vi "Beta Ver 1.1.vi"() -> ()   [LabVIEW 2015]
uses:
  <instrlib>/Keithley 622x LV 2009/Configure/Source/Typedefs/KE622x -- Current Range.ctl
  <instrlib>/Keithley 622x LV 2009/Configure/Source/Typedefs/KE622x -- Current Ranges.ctl
  <instrlib>/Keithley 622x LV 2009/Typedefs/KE622x -- On Off Control.ctl
  <instrlib>/Keithley 622x LV 2009/Utility/Typedefs/KE622x -- Instrument Type.ctl
  <instrlib>/Keithley 622x LV 2009/Configure/Source/Typedefs/KE622x -- Voltage Limit.ctl
  <instrlib>/Keithley 2000/Public/Configure/Configure DC Volts.vi
  <userlib>/LV-Link3/PolySubVIs/DtCreateAinChan.vi
  <userlib>/LV-Link3/PolySubVIs/DtOLReadMultipleSingle.vi
  <instrlib>/Keithley 2000/Keithley 2000.lvlib
  <instrlib>/Keithley 622x LV 2009/Keithley 622x.lvlib
panel:
  in  "Setup":u16(ring) items=["START, STOP, STEP, CONFIGURATION", "PRINCETON LOCK-IN AMP"]
  out "prev_time_const":i32
  out "prev_range":i32
  out "XTC":i32
  out "SEN":i32
  in  "Time Delay":u16(ring) items=["0.1", "1", "3", "10", "30", "60"]
  out "FILE":refnum<file>
  out "Tick":u32
  in  "MULTIPLE GRAPHS Y":u16(ring) items=["Linear", "Log"]
  in  "MULTIPLE GRAPHS X":u16(ring) items=["Linear", "Log"]
  in  "TIME GRAPH Y":u16(ring) items=["Linear", "Log"]
  in  "TIME GRAPH X":u16(ring) items=["Linear", "Log"]
  in  "Lock-In, Y":dbl=1.0
  in  "Lock-In, X":dbl=1.0
  in  "DAQ A4":dbl=1.0
  in  "DAQ A3":dbl=1.0
  in  "DAQ A2":dbl=1.0
  in  "DAQ A1":dbl=1.0
  in  "DAQ A0":dbl=1.0
  in  "2000":dbl=1.0
  in  "Current":dbl=1000.0
  in  "Display Type 3":u16(ring)=3 items=["X %", "Y %", "X Calibrated", "Y Calibrated", "Mag %", "Mag Calibrated", "Phase Degrees", "Ratio", "ADC 1", "ADC 2", "ADC 3", "ADC 4 ", "Noise %", "Noise Calibrated", "Ref Frequency", "", ""]
  in  "Display Type 2":u16(ring)=2 items=["X %", "Y %", "X Calibrated", "Y Calibrated", "Mag %", "Mag Calibrated", "Phase Degrees", "Ratio", "ADC 1", "ADC 2", "ADC 3", "ADC 4 ", "Noise %", "Noise Calibrated", "Ref Frequency", "", ""]
  out "Units 3":string
  out "Display 3":dbl format="%.3f"
  out "Units 2":string
  out "Display 2":dbl format="%.3f"
  out "DAQ A4":dbl format="%#_13g"
  out "DAQ_clust":T1
  out "DAQ A3":dbl format="%#_13g"
  out "DAQ A2":dbl format="%#_13g"
  out "DAQ A1":dbl format="%#_13g"
  out "Real stop cur":dbl format="%#_13g"
  out "Real start cur":dbl format="%#_13g"
  in  "Stop cur prefix":u16(ring)=2
  in  "Start cur prefix":u16(ring)=2
  out "MULTIPLE GRAPHS":cluster{dbl[], dbl[]}[](graph)
  in  "X-Axis":T2(ring)
  in  "Range":u8(ring)=20 items=["100nV", "200nV", "500nV", "1µV", "2µV", "5µV", "10µV", "20µV", "50µV", "100µV", "200µV", "500µV", "1mV", "2mV", "5mV", "10mV", "20mV", "50mV", "100mV", "200mV", "500mV", "1V"]
  in  "Display Type copy":u16(ring)=3 items=["X %", "Y %", "X Calibrated", "Y Calibrated", "Mag %", "Mag Calibrated", "Phase Degrees", "Ratio", "ADC 1", "ADC 2", "ADC 3", "ADC 4 ", "Noise %", "Noise Calibrated", "Ref Frequency", "", ""]
  out "Units copy":string
  out "Display copy":dbl format="%.3f"
  out "Overload":bool
  out "Display":dbl format="%.3f"
  out "Units":string
  in  "Display Type":u16(ring)=2 items=["X %", "Y %", "X Calibrated", "Y Calibrated", "Mag %", "Mag Calibrated", "Phase Degrees", "Ratio", "ADC 1", "ADC 2", "ADC 3", "ADC 4 ", "Noise %", "Noise Calibrated", "Ref Frequency", "", ""]
  in  "Time Constant":u16(ring)=7 items=["MIN", "1ms", "3ms", "10ms", "30ms", "100ms", "300ms", "1s", "3s", "10s", "30s", "100s", "300s"]
  in  "Slope":u8(ring) items=["6db/octave", "12dB/octave"]
  in  "Dynamic Reserve":u16(ring)=1 items=["High Stability", "Normal", "High Reserve"]
  in  "Auto Sensitivity":bool
  in  "Auto Measure":bool
  out "6221_error_out":errorcluster
  out "2000_error_out":errorcluster
  out "5110_error_out":errorcluster
  out "Input Mode":i32(ring) items=[" Voltage Input (A or A-B) ", "Current Input 10E6 V/A", "Current Input 10E8 V/A"]
  out "5110":refnum<visa-resource-name>
  in  "GPIB Address":i8=11 min=1 max=32 step=1
  out "DAQ A0":dbl format="%#_13g"
  out "2000":dbl format="%#_13g"
  in  "Device":string(combo)
  in  "Number \nof points":i32=10
  in  "Folder\nprename":string
  out "TIME GRAPH":cluster{dbl[], dbl[]}[](graph)
  out "T0":u32
  out "LIMIT":bool
  out "LIMIT":bool
  out "Error Code":string
  in  "Comments":string
  out "2000":refnum<visa-resource-name>
  out "6221":refnum<visa-resource-name>
  out "Step  (A)":dbl=5e-05 format="%#_3p"
  in  "Stop\ncurrent (A)":dbl=2.0 format="%#_6p"
  in  "Start \ncurrent (A)":dbl=1.0 format="%#_6p"
  in  "Check For SCPI Errors? (T)":bool=TRUE
  out "Interlock Tripped?":bool
  out "Compliance?":bool
  in  "Turn Off Output \nIf Compliance?":bool=TRUE
  in  "Turning ON/OFF\ncurrent output":T3=enum."On"
  in  "Range Selection":T4={"Auto Range?"=TRUE, "Man / Selected\nRange"=enum."2nA"}
  # "FILE CONFIGURATION"
  # "ADMIN PANEL"
  # "MULTIPLIERS"
  # "SCALES"
  # "KEITHLEY 6221 CONFIGURATION (ADMIN ONLY)"
  # "KEITHLEY DAQ CONFIGURATION (ADMIN ONLY)"
  # "PRINCETON LOCK-IN AMP (ADMIN ONLY)"
  # "I don't know what the hell it is,\njust don't touch it"
  # "INPUT CONFIGURATION"
  # "READINGS"
  # "IF ON"
  # "Compliance = Limiting output voltage\nThis switch determines if we want to switch \noff the current output if wee exceed compliance"
  # "SCALES"
  # "There is a safe switch at \nthe back of the instrument \nThis indicator shows if it is on"
  # "You have hit a damn jackpot \nby exceeding the limited voltage\nCongrats"
  # "LOCK-IN READINGS"
  # "RIGHT DISPLAY"
  # "LEFT DISPLAY"
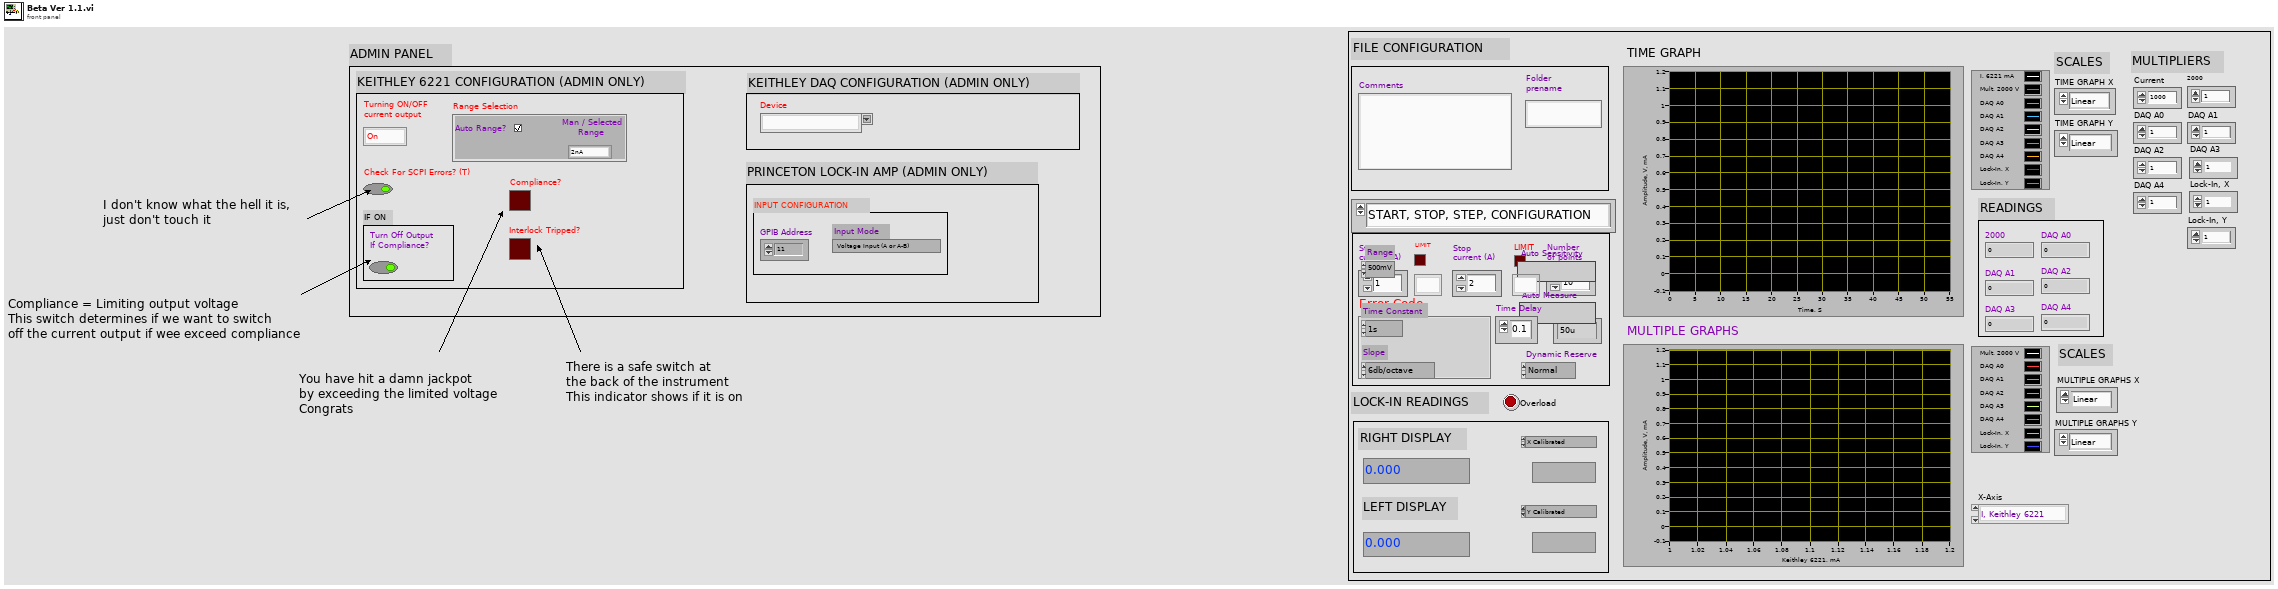
[diagram p1: front panel]
types:
  T1 = cluster{"Task out":i32, "Actual Number of Channels":u32, "error out":errorcluster}
  T2 = enum16{"I, Keithley 6221", "V, Keithley 2000", "V, Keithley DAQ A0", "V, Keithley DAQ A1", "V, Keithley DAQ A2", "V, Keithley DAQ A3", "V, Keithley DAQ A4", "V, Lock-In X", "V, Lock-In Y"}
  T3 = typedef "Keithley 622x.lvlib/KE622x -- On Off Control.ctl" = enum16{"Off", "On"}
  T4 = typedef "Keithley 622x.lvlib/KE622x -- Current Range.ctl" = cluster{"Auto Range?":bool, "Man / Selected\nRange":T5}
  T5 = typedef "Keithley 622x.lvlib/KE622x -- Current Ranges.ctl" = enum16{"2nA", "20nA", "200nA", "2uA", "20uA", "200uA", "2mA", "20mA", "100mA"}
  T6 = typedef "Keithley 622x.lvlib/KE622x -- Instrument Type.ctl" = enum16{"KE6220", "KE6221"}
  T7 = typedef "Keithley 622x.lvlib/KE622x -- Voltage Limit.ctl" = dbl
  T8 = cluster{dbl[], dbl[], dbl[], dbl[], dbl[], dbl[], dbl[], dbl[], dbl[], dbl[]}
  T9 = cluster{"5110":refnum<visa-resource-name>, "2000":refnum<visa-resource-name>, "6221":refnum<visa-resource-name>, "5110_error_out":errorcluster, "6221_error_out":errorcluster, "2000_error_out":errorcluster, "DAQ_clust":cluster{"Task out":i32, "Actual Number of Channels":u32, "error out":errorcluster}}
  T10 = cluster{dbl, dbl, dbl, dbl, dbl, "Measurement":dbl}
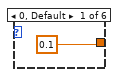
[diagram p2: hidden frame]
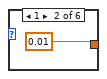
[diagram p3: hidden frame]
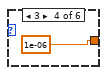
[diagram p4: hidden frame]
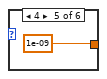
[diagram p5: hidden frame]
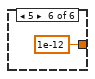
[diagram p6: hidden frame]
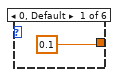
[diagram p7: hidden frame]
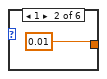
[diagram p8: hidden frame]
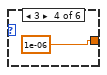
[diagram p9: hidden frame]
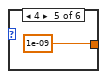
[diagram p10: hidden frame]
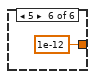
[diagram p11: hidden frame]
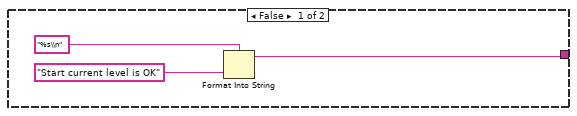
[diagram p12: hidden frame]
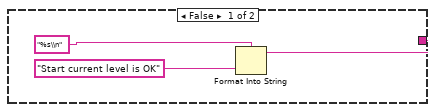
[diagram p13: hidden frame]
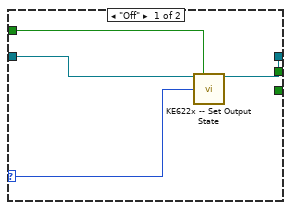
[diagram p14: hidden frame]
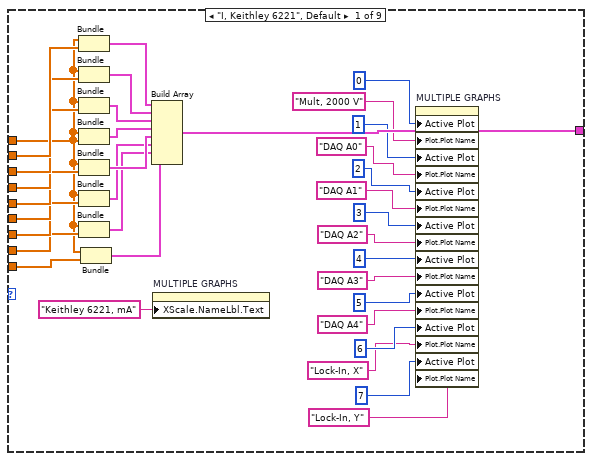
[diagram p15: hidden frame]
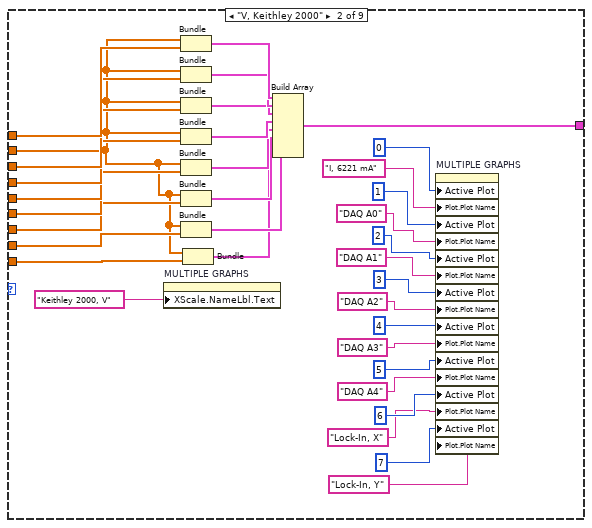
[diagram p16: hidden frame]
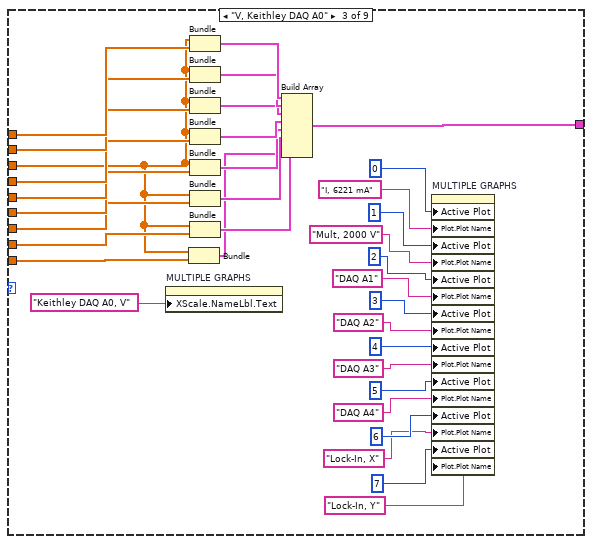
[diagram p17: hidden frame]
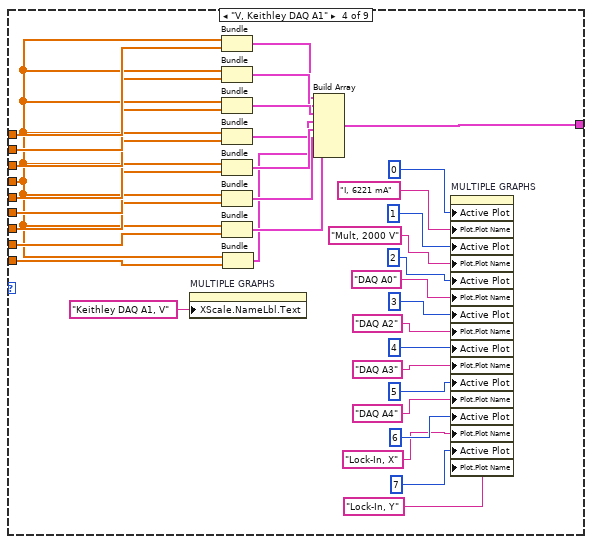
[diagram p18: hidden frame]
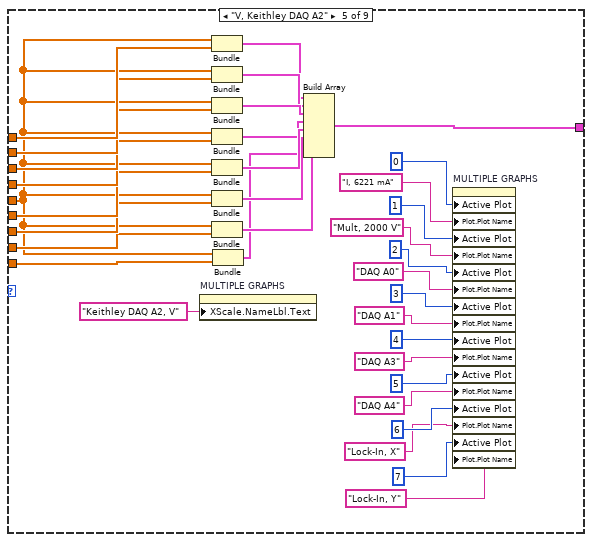
[diagram p19: hidden frame]
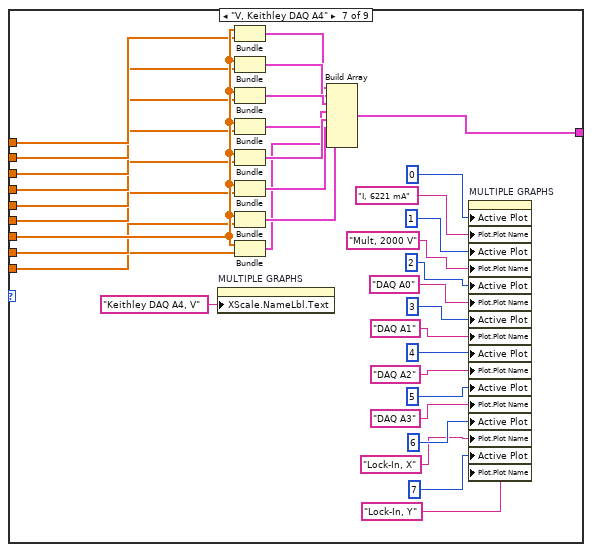
[diagram p20: hidden frame]
diagram:
  n1 = flat-sequence {
    tunnel: [w153] -> w1
    tunnel: w1 -> [w942]
    frame #0 {
      w16 = TRUE  # reset
      w17 = FALSE  # ID query
      # "Initialize Keithley DAQ \n(getting board name)"
      # "Initialize Lock-In 5110"
      # "Initialize Keithley 2000"
      # "Initialize Keithley 6221"
      n2 = call <userlib>:"DtOLGetBoardNames.vi"() -> ("Number of boards"=w2:u32)  [unwired: 9 in, 2 out]
      n3 = Initialize Array("", w2) -> (w4:string[])
      n4 = call <instrlib>:"Initialize.vi"("VISA resource name"=refnum<visa-resource-name> "KEITHLEY_MULTIMETER") -> ("VISA resource name out"=w12:refnum<visa-resource-name>)  [unwired: 17 in, 1 out]
      n5 = for {
        N: w2 -> [_]
        shift-right: [w26] -> w7
        shift-left: w4 -> [w27]
        i -> [w25]
        n6 = Add(x=1, y=w25) -> (x+y=w29:i32)
        n7 = call <userlib>:"DtOLGetBoardNames.vi"("Select Board"=w29) -> ("Board Name"=w24:string)  [unwired: 8 in, 2 out]
        n8 = Replace Array Subset(array=w27, new element=w24, index=w25) -> (w26:string[])
      }
      n9 = call <instrlib>:"Initialize.vi"("VISA resource name"=refnum<visa-resource-name> "KEITHLEY_DC_AC_CURRENT_SOURCE", "Error Queue Option"=enum16{"Clear Error Queue", "Error Query"}."Clear Error Queue", "Instrument Type"=KE622x_--_Instrument_Type."KE6221") -> ("VISA resource name out"=→"6221":refnum<visa-resource-name>, "error out"=→"6221_error_out":errorcluster)  [unwired: 11 in]
      n10 = call-poly <instrlib>:"Configure Measurement.vi"("VISA resource name"=w12) -> ("VISA resource name out"=→"2000":refnum<visa-resource-name>, "error out"=→"2000_error_out":errorcluster)  [unwired: 17 in]
      n11 = call "SR51XX Initialize"("VISA session (for class)"=refnum<visa-resource-name> "LOCK_IN_5110_PRINCETON", "Interface"=FALSE, "ID query"=w17, "GPIB Address"="GPIB Address", "reset"=w16) -> ("VISA session"=→"5110":refnum<visa-resource-name>, "error out"=→"5110_error_out":errorcluster)  [unwired: 8 in, 1 out]
      n12 = Index Array(array=w7, index=0) -> (element=w6:string)
      n13 = property on="Device" class="CmbBox"("Strings[]"=w7, "Value"=w6) -> ()  [unwired: 2 in, 2 out]
    }
    frame #1 {
      # "Putting in a loop \ninstead of \"STOP\""
      n14 = case shown="2" "Start cur prefix" {
        tunnel: [0.1 0.01 0.001 1e-06 1e-09 1e-12] -> w39
        frame 0, Default {
        }
        frame 1 {
        }
        frame 2 {
        }
        frame 3 {
        }
        frame 4 {
        }
        frame 5 {
        }
      }
      n15 = case shown="2" "Stop cur prefix" {
        tunnel: [0.1 0.01 0.001 1e-06 1e-09 1e-12] -> w41
        frame 0, Default {
        }
        frame 1 {
        }
        frame 2 {
        }
        frame 3 {
        }
        frame 4 {
        }
        frame 5 {
        }
      }
      n16 = Multiply(x=w39, y="Start \ncurrent (A)") -> (x*y=w43:dbl)
      "Real start cur" <- w43
      n17 = Multiply(x=w41, y="Stop\ncurrent (A)") -> (x*y=w44:dbl)
      "Real stop cur" <- w44
      n18 = Greater?(x=w44, y=T7 0.01) -> (0:w33:bool)
      n19 = Greater?(x=w43, y=T7 0.01) -> (0:w34:bool)
      n20 = case shown="True" w33 {
        selector: w33 -> [_ w60]
        tunnel: [w57 w63] -> w31
        frame False {
          n21 = Format Into String(format string="%s\\n", "Start current level is OK" ("false string")) -> (resulting string=w57:string)  [unwired: 2 in, 1 out]
        }
        frame True {
          n22 = flat-sequence {
            tunnel: [w65] -> w62
            tunnel: [w64] -> w61
            tunnel: w60 -> [w64]
            tunnel: [w69] -> w63
            tunnel: w62 -> [w69]
            tunnel: w61 -> [w70]
            frame #0 {
              n23 = Format Into String(format string="%s\\n%s\\n", "Stop current level" ("String"), "exceeded the  limit: 10mA" ("input 2")) -> (resulting string=w65:string)  [unwired: 2 in, 1 out]
            }
            frame #1 {
              n24 = while {
                tunnel: w70 -> [w71]
                stop <- w71 continue-if-true
                "LIMIT" <- w71
              }
              n25 = property on="Error Code" class="Str"("Text.Text"=w69) -> ()  [unwired: 2 in, 2 out]
            }
          }
        }
      }
      n26 = case shown="True" w34 {
        selector: w34 -> [_ w76]
        tunnel: [w72 w78] -> w32
        frame False {
          n27 = Format Into String(format string="%s\\n", "Start current level is OK" ("false string")) -> (resulting string=w72:string)  [unwired: 2 in, 1 out]
        }
        frame True {
          n28 = flat-sequence {
            tunnel: [w80] -> w77
            tunnel: w76 -> [w79]
            tunnel: [w79] -> w75
            tunnel: [w84] -> w78
            tunnel: w77 -> [w84]
            tunnel: w75 -> [w85]
            frame #0 {
              n29 = Format Into String(format string="%s\\n%s\\n", "Start current level" ("String"), "exceeded the limit: 10mA" ("input 2")) -> (resulting string=w80:string)  [unwired: 2 in, 1 out]
            }
            frame #1 {
              n30 = while {
                tunnel: w85 -> [w86]
                stop <- w86 continue-if-true
                "LIMIT" <- w86
              }
              n31 = property on="Error Code" class="Str"("Text.Text"=w84) -> ()  [unwired: 2 in, 2 out]
            }
          }
        }
      }
      n32 = Concatenate Strings(w32, w31) -> (→"Error Code":string)
    }
    frame #2 {
      # "Calculating steps by number\nof points"
      n33 = local read "Real stop cur"() -> (w88:dbl)
      n34 = local read "Real start cur"() -> (w89:dbl)
      n35 = Subtract(x=w88, y=w89) -> (x-y=w91:dbl)
      n36 = Divide(x=w91, y="Number \nof points") -> (x/y=→"Step  (A)":dbl)
    }
    frame #3 {
      # "Adding headlines"
      # "Creating folder&file"
      # "Creating comments"
      # "Writing instr params"
      n37 = local read "5110"() -> (w104:refnum<visa-resource-name>)
      n38 = local read "Real stop cur"() -> (w102:dbl)
      n39 = local read "Real start cur"() -> (w103:dbl)
      n40 = call "folder_creation.vi"("Name"="Folder\nprename") -> ("String"=w95:string)
      n41 = call "file_creation.vi"("String"=w95) -> ("refnum out"=w101:refnum<file>)
      "FILE" <- w101
      n42 = call "com_inst.vi"("Stop current"=w102, "Start current"=w103, "VISA session (for class)"=w104) -> ("XTC"=w106:i32, "SEN"=w105:i32, "concatenated string"=w107:string)
      "SEN" <- w105
      "XTC" <- w106
      n43 = Format Into String(format string="# %s\\n", initial string=w101, "Comments") -> (resulting string=w99:refnum<file>)  [unwired: 1 in, 1 out]
      n44 = property on="Time Constant" class="Ring (strict)"("Value"=w106) -> ()  [unwired: 2 in, 2 out]
      n45 = Format Into String(format string="# %s\\n", initial string=w99, w107) -> (resulting string=w100:refnum<file>)  [unwired: 1 in, 1 out]
      n46 = property on="Range" class="Ring (strict)"("Value"=w105) -> ()  [unwired: 2 in, 2 out]
      n47 = Format Into String(format string="# %-6s  %-12s %-12s %-14s %-12s %-14s %-12s %-12s %-14s%-14s\\n", initial string=w100, "t, ms" ("input 3"), "6221, A" ("input 3"), "2000, V" ("input 1"), "5110_X, V" ("input 3"), "5110_Y, V " ("input 3"), "DAQ A0, V" ("input 2"), "DAQ A1, V" ("input 2"), "DAQ A2, V" ("input 2"), "DAQ A3, V" ("input 2"), "DAQ A4, V" ("input 2")) -> ()  [unwired: 1 in, 2 out]
    }
    frame #4 {
      # "Variables"
      # "Time Intit"
      n48 = property on="SEN" class="DigNum (strict)"() -> ("Value"=→"prev_range":i32)  [unwired: 2 in, 2 out]
      n49 = property on="XTC" class="DigNum (strict)"() -> ("Value"=→"prev_time_const":i32)  [unwired: 2 in, 2 out]
      n50 = Wait Until Next ms Multiple(millisecond multiple=u32 1000) -> (millisecond timer value=→"T0":u32)
    }
    frame #5 {
      n51 = flat-sequence {
        tunnel: [w131] -> w121
        tunnel: [w149] -> _
        tunnel: [w151] -> _
        tunnel: w121 -> [w150]
        frame #0 {
          # "Current range \nselection check"
          # "Checking for compliance\nand interlock errors"
          n52 = local read "6221"() -> (w134:refnum<visa-resource-name>)
          n53 = call <instrlib>:"KE622x -- Set Current Range.vi"("Resource In"=w134, "Current Range In"="Range Selection", "Read Back Set Values? (T)"=FALSE) -> ("Resource Out (dupl)"=w139:refnum<visa-resource-name>)  [unwired: 10 in, 2 out]
          n54 = case shown="\"On\"" "Turning ON/OFF\ncurrent output" {
            selector: "Turning ON/OFF\ncurrent output" -> [w143 _]
            tunnel: [_ w147] -> w137
            tunnel: [_ w146] -> w138
            tunnel: "Check For SCPI Errors? (T)" -> [w142 _]
            tunnel: w139 -> [w140 w145]
            tunnel: [w141 w144] -> w131
            frame "Off" {
              n55 = call <instrlib>:"KE622x -- Set Output State.vi"("Resource In"=w140, "Check For SCPI Errors? (T)"=w142, "Output State"=w143) -> ("Resource Out (dupl)"=w141:refnum<visa-resource-name>)  [unwired: 11 in, 1 out]
            }
            frame "On" {
              n56 = call <instrlib>:"KE622x -- Turn Output On And Check For Errors.vi"("Resource In"=w145, "Turn Off Output If Compliance?"="Turn Off Output \nIf Compliance?") -> ("Resource Out (dupl)"=w144:refnum<visa-resource-name>, "Interlock Tripped?"=w147:bool, "Compliance?"=w146:bool)  [unwired: 10 in, 1 out]
            }
          }
          "Interlock Tripped?" <- w137
          "Compliance?" <- w138
        }
        frame #1 {
          # "Setting start current"
          n57 = local read "Real start cur"() -> (w149:dbl)
          n58 = Wait (ms)(milliseconds to wait=u32 100) -> ()  [unwired: 1 out]
          n59 = call <instrlib>:"KE622x -- Set Current Level.vi"("Resource In"=w150, "Current Level (A) In"=w149) -> ("Resource Out (dupl)"=w151:refnum<visa-resource-name>)  [unwired: 12 in, 1 out]
        }
      }
      n60 = flat-sequence {
        frame #0 {
          w126 = 100 items=["SingleEnded"=100, "Differential"=101] ("Channel Type")
          # "Configure the input channel"
          n61 = call-poly <userlib>:"DtOLCreateTask.vi"("Channel Type"=w126, "Range Min"=-10.0, "Range Max"=10.0, "Board Name"="Device", "Channel"="0:4" ("Channels")) -> ("Task out"=w125:i32, "Actual Number of Channels"=w124:u32, "error out"=w123:errorcluster)  [unwired: 8 in]
          n62 = Bundle("Task out"=w125, "Actual Number of Channels"=w124, "error out"=w123) -> (→"DAQ_clust":T1)  [unwired: 1 in]
        }
      }
    }
    frame #6 {
      # "V, DAQ A4"
      # "V, DAQ A3"
      # "V, DAQ A2"
      # "V, DAQ A1"
      # "Y-V, 5110"
      # "X-V, 5110"
      # "I, 6221"
      # "Time"
      # "V, DAQ A0"
      # "V, 2000"
      n63 = local read "5110"() -> (w164:refnum<visa-resource-name>)
      n64 = local read "2000"() -> (w163:refnum<visa-resource-name>)
      n65 = local read "6221"() -> (w162:refnum<visa-resource-name>)
      n66 = local read "5110_error_out"() -> (w161:errorcluster)
      n67 = local read "6221_error_out"() -> (w160:errorcluster)
      n68 = local read "2000_error_out"() -> (w159:errorcluster)
      n69 = local read "DAQ_clust"() -> (w158:T1)
      n70 = while {
        shift-right: [w362] -> _
        shift-left: dbl[] [] -> [w214]
        shift-right: [w363] -> _
        shift-left: i32[] [] -> [w215]
        tunnel: w163 -> [w190]
        tunnel: w162 -> [w189]
        shift-right: [w335] -> _
        shift-left: dbl[] [] -> [w210]
        tunnel: w164 -> [w191]
        tunnel: w161 -> [w188]
        tunnel: w160 -> [w187]
        tunnel: w159 -> [w186]
        shift-right: [w337] -> _
        shift-left: dbl[] [] -> [w208]
        shift-right: [w338] -> _
        shift-left: dbl[] [] -> [w207]
        shift-right: [w364] -> _
        shift-left: dbl[] [] -> [w216]
        tunnel: w158 -> [w185]
        shift-right: [w361] -> _
        shift-left: dbl[] [] -> [w213]
        shift-right: [w360] -> _
        shift-left: dbl[] [] -> [w212]
        shift-right: [w359] -> _
        shift-left: dbl[] [] -> [w211]
        shift-right: [w336] -> _
        shift-left: dbl[] [] -> [w209]
        tunnel: [w192] -> w153
        i -> [w389]
        stop <- w397 stop-if-true
        n71 = Bundle(w216, w215, w214, w213, w212, w211, w210, w209, w208, w207) -> (w203:T8)  [unwired: 1 in]
        n72 = Quotient & Remainder(x=w389, y=10) -> (floor(x/y)=w394:i32)  [unwired: 1 out]
        n73 = Equal?(x=0, y=w389) -> (x = y?=w391:bool)
        n74 = Bundle("5110"=w191, "2000"=w190, "6221"=w189, "5110_error_out"=w188, "6221_error_out"=w187, "2000_error_out"=w186, "DAQ_clust"=w185) -> (w183:T9)  [unwired: 1 in]
        n75 = Equal?(x=1, y=w394) -> (x = y?=w390:bool)
        n76 = flat-sequence {
          tunnel: w391 -> [w718]
          tunnel: [w718] -> w378
          tunnel: w390 -> [w717]
          tunnel: [w717] -> w376
          tunnel: [w716] -> w388
          tunnel: [w715] -> w184
          tunnel: w183 -> [w715]
          tunnel: w378 -> [w722]
          tunnel: [w722] -> w377
          tunnel: w376 -> [w721]
          tunnel: [w721] -> w375
          tunnel: w184 -> [w719]
          tunnel: [w719] -> w182
          tunnel: [w733] -> w387
          tunnel: [w732] -> w386
          tunnel: w377 -> [w731]
          tunnel: [w731] -> w385
          tunnel: w375 -> [w730]
          tunnel: w182 -> [w729]
          tunnel: [w729] -> w181
          tunnel: w387 -> [w756]
          tunnel: [w755] -> w253
          tunnel: w386 -> [w754]
          tunnel: [w753] -> w251
          tunnel: w385 -> [w751]
          tunnel: [w751] -> w249
          tunnel: ["Auto Measure"] -> w247
          tunnel: ["Auto Sensitivity"] -> w245
          tunnel: [w746] -> w243
          tunnel: w181 -> [w743]
          tunnel: [w743] -> w178
          tunnel: w253 -> [w758]
          tunnel: [w758] -> w252
          tunnel: w251 -> [w766]
          tunnel: [w766] -> w250
          tunnel: w249 -> [w765]
          tunnel: [w765] -> w248
          tunnel: w247 -> [w764]
          tunnel: [w764] -> w246
          tunnel: w245 -> [w763]
          tunnel: [w763] -> w244
          tunnel: w243 -> [w762]
          tunnel: [w762] -> w242
          tunnel: [w757] -> w179
          tunnel: w178 -> [w757]
          tunnel: w252 -> [w785]
          tunnel: w250 -> [w783]
          tunnel: [w782] -> w227
          tunnel: w248 -> [w789]
          tunnel: [w789] -> w229
          tunnel: w246 -> [w787]
          tunnel: [w787] -> w231
          tunnel: w244 -> [w788]
          tunnel: [w788] -> w233
          tunnel: w242 -> [w778]
          tunnel: [w778] -> w235
          tunnel: [w784] -> w237
          tunnel: ["Time Constant"] -> w239
          tunnel: ["Slope"] -> w241
          tunnel: [w775] -> w180
          tunnel: w179 -> [w775]
          tunnel: w241 -> [w801]
          tunnel: [w801] -> w240
          tunnel: w239 -> [w800]
          tunnel: [w800] -> w238
          tunnel: w237 -> [w793]
          tunnel: [w793] -> w236
          tunnel: w235 -> [w799]
          tunnel: [w799] -> w234
          tunnel: w233 -> [w798]
          tunnel: [w798] -> w232
          tunnel: w231 -> [w797]
          tunnel: [w797] -> w230
          tunnel: w229 -> [w796]
          tunnel: [w796] -> w228
          tunnel: w227 -> [w795]
          tunnel: [w795] -> w226
          tunnel: w180 -> [w790]
          tunnel: [w790] -> w174
          tunnel: [w816] -> w333
          tunnel: [w827] -> w332
          tunnel: [w826] -> w331
          tunnel: [w825] -> w330
          tunnel: [w818] -> w329
          tunnel: [w821] -> w328
          tunnel: [w819] -> w327
          tunnel: [w824] -> w326
          tunnel: w240 -> [w824]
          tunnel: w238 -> [w819]
          tunnel: w236 -> [w822]
          tunnel: w234 -> [w818]
          tunnel: w232 -> [w825]
          tunnel: w230 -> [w826]
          tunnel: w228 -> [w827]
          tunnel: w226 -> [w817]
          tunnel: [w810] -> w175
          tunnel: w174 -> [w810]
          tunnel: w333 -> [w842]
          tunnel: [w841] -> w325
          tunnel: w332 -> [w846]
          tunnel: [w846] -> w323
          tunnel: w331 -> [w845]
          tunnel: [w845] -> w321
          tunnel: w330 -> [w844]
          tunnel: [w844] -> w319
          tunnel: w329 -> [w836]
          tunnel: [w836] -> w317
          tunnel: w328 -> [w843]
          tunnel: [w840] -> w315
          tunnel: w327 -> [w838]
          tunnel: [w838] -> w313
          tunnel: w326 -> [w835]
          tunnel: [w835] -> w311
          tunnel: [w831] -> w308
          tunnel: [w828] -> w176
          tunnel: w175 -> [w828]
          tunnel: w325 -> [w860]
          tunnel: [w859] -> w324
          tunnel: w323 -> [w865]
          tunnel: [w865] -> w322
          tunnel: w321 -> [w864]
          tunnel: [w864] -> w320
          tunnel: w319 -> [w863]
          tunnel: [w863] -> w318
          tunnel: w317 -> [w855]
          tunnel: [w855] -> w316
          tunnel: w315 -> [w862]
          tunnel: [w861] -> w314
          tunnel: w313 -> [w857]
          tunnel: [w857] -> w312
          tunnel: w311 -> [w854]
          tunnel: [w854] -> w310
          tunnel: [w850] -> w309
          tunnel: [w847] -> w177
          tunnel: w176 -> [w847]
          tunnel: w324 -> [w874]
          tunnel: w322 -> [w884]
          tunnel: [w884] -> w384
          tunnel: w320 -> [w883]
          tunnel: [w883] -> w383
          tunnel: w318 -> [w882]
          tunnel: [w882] -> w382
          tunnel: w316 -> [w875]
          tunnel: w314 -> [w873]
          tunnel: w312 -> [w876]
          tunnel: w310 -> [w877]
          tunnel: [w872] -> w381
          tunnel: w177 -> [w867]
          tunnel: [w866] -> w172
          tunnel: w389 -> [w890]
          tunnel: [w887] -> w397
          tunnel: [w886] -> w398
          tunnel: [w886] -> w372
          tunnel: w381 -> [_]
          tunnel: w382 -> [_]
          tunnel: w383 -> [_]
          tunnel: w384 -> [_]
          tunnel: [w885] -> w173
          tunnel: w172 -> [w885]
          tunnel: w398 -> [w900]
          tunnel: w173 -> [w896]
          tunnel: [w893] -> w171
          tunnel: [w933] -> w396
          tunnel: [w931] -> w347
          tunnel: [w932] -> w346
          tunnel: [w933] -> w342
          tunnel: [w930] -> w345
          tunnel: [w929] -> w344
          tunnel: [w928] -> w343
          tunnel: [w901] -> w192
          tunnel: w171 -> [w906]
          frame #0 {
            n77 = Tick Count (ms)() -> (millisecond timer value=w716:u32)
            "Tick" <- w716
          }
          frame #1 {
            n78 = case shown="1" "Setup" {
              frame 0, Default {
                n79 = flat-sequence {
                  frame #0 {
                    w723 = FALSE ("Visible")
                    n80 = property on="Slope" class="Ring (strict)"("Visible"=w723) -> ()  [unwired: 2 in, 2 out]
                    n81 = property on="Range" class="Ring (strict)"("Visible"=w723) -> ()  [unwired: 2 in, 2 out]
                    n82 = property on="Time Constant" class="Ring (strict)"("Visible"=w723) -> ()  [unwired: 2 in, 2 out]
                    n83 = property on="Dynamic Reserve" class="Ring (strict)"("Visible"=w723) -> ()  [unwired: 2 in, 2 out]
                    n84 = property on="Auto Sensitivity" class="Bool (strict)"("Visible"=w723) -> ()  [unwired: 2 in, 2 out]
                    n85 = property on="Auto Measure" class="Bool (strict)"("Visible"=w723) -> ()  [unwired: 2 in, 2 out]
                  }
                  frame #1 {
                    w724 = TRUE ("Visible")
                    n86 = property on="Start \ncurrent (A)" class="DigNum (strict)"("Visible"=w724) -> ()  [unwired: 2 in, 2 out]
                    n87 = property on="Stop\ncurrent (A)" class="DigNum (strict)"("Visible"=w724) -> ()  [unwired: 2 in, 2 out]
                    n88 = property on="LIMIT" class="Bool (strict)"("Visible"=w724) -> ()  [unwired: 2 in, 2 out]
                    n89 = property on="LIMIT" class="Bool (strict)"("Visible"=w724) -> ()  [unwired: 2 in, 2 out]
                    n90 = property on="Start cur prefix" class="Ring (strict)"("Visible"=w724) -> ()  [unwired: 2 in, 2 out]
                    n91 = property on="Stop cur prefix" class="Ring (strict)"("Visible"=w724) -> ()  [unwired: 2 in, 2 out]
                    n92 = property on="Step  (A)" class="DigNum (strict)"("Visible"=w724) -> ()  [unwired: 2 in, 2 out]
                    n93 = property on="Number \nof points" class="DigNum (strict)"("Visible"=w724) -> ()  [unwired: 2 in, 2 out]
                    n94 = property on="Time Delay" class="Ring (strict)"("Visible"=w724) -> ()  [unwired: 2 in, 2 out]
                    n95 = property on="Error Code" class="Str"("Visible"=w724) -> ()  [unwired: 2 in, 2 out]
                  }
                }
              }
              frame 1 {
                n96 = flat-sequence {
                  frame #0 {
                    w725 = TRUE ("Visible")
                    n97 = property on="Slope" class="Ring (strict)"("Visible"=w725) -> ()  [unwired: 2 in, 2 out]
                    n98 = property on="Range" class="Ring (strict)"("Visible"=w725) -> ()  [unwired: 2 in, 2 out]
                    n99 = property on="Time Constant" class="Ring (strict)"("Visible"=w725) -> ()  [unwired: 2 in, 2 out]
                    n100 = property on="Dynamic Reserve" class="Ring (strict)"("Visible"=w725) -> ()  [unwired: 2 in, 2 out]
                    n101 = property on="Auto Sensitivity" class="Bool (strict)"("Visible"=w725) -> ()  [unwired: 2 in, 2 out]
                    n102 = property on="Auto Measure" class="Bool (strict)"("Visible"=w725) -> ()  [unwired: 2 in, 2 out]
                  }
                  frame #1 {
                    w726 = FALSE ("Visible")
                    n103 = property on="Start \ncurrent (A)" class="DigNum (strict)"("Visible"=w726) -> ()  [unwired: 2 in, 2 out]
                    n104 = property on="Stop\ncurrent (A)" class="DigNum (strict)"("Visible"=w726) -> ()  [unwired: 2 in, 2 out]
                    n105 = property on="LIMIT" class="Bool (strict)"("Visible"=w726) -> ()  [unwired: 2 in, 2 out]
                    n106 = property on="LIMIT" class="Bool (strict)"("Visible"=w726) -> ()  [unwired: 2 in, 2 out]
                    n107 = property on="Start cur prefix" class="Ring (strict)"("Visible"=w726) -> ()  [unwired: 2 in, 2 out]
                    n108 = property on="Stop cur prefix" class="Ring (strict)"("Visible"=w726) -> ()  [unwired: 2 in, 2 out]
                    n109 = property on="Step  (A)" class="DigNum (strict)"("Visible"=w726) -> ()  [unwired: 2 in, 2 out]
                    n110 = property on="Number \nof points" class="DigNum (strict)"("Visible"=w726) -> ()  [unwired: 2 in, 2 out]
                    n111 = property on="Time Delay" class="Ring (strict)"("Visible"=w726) -> ()  [unwired: 2 in, 2 out]
                    n112 = property on="Error Code" class="Str"("Visible"=w726) -> ()  [unwired: 2 in, 2 out]
                  }
                }
              }
            }
          }
          frame #2 {
            n113 = Unbundle By Name(w729) -> ("5110"=w728:refnum<visa-resource-name>, "5110_error_out"=w727:errorcluster)
            n114 = case shown="True" w730 {
              tunnel: w728 -> [w737 w742]
              tunnel: [w736 w740] -> w735
              tunnel: [w737 w739] -> w734
              tunnel: w727 -> [w736 w738]
              frame False {
              }
              frame True {
                n115 = call "SR51XX Read Preamp Input Mode"("VISA session (for class)"=w742, "error in (no error)"=w738) -> ("VISA session"=w739:refnum<visa-resource-name>, "Input Mode"=w741:i32, "error out"=w740:errorcluster)  [unwired: 15 in]
                n116 = local write "Input Mode"(w741) -> ()
              }
            }
            n117 = call "SR51XX Configure Signal Channel Input"("VISA session (for class)"=w734, "error in (no error)"=w735, "Update"=w731) -> ("VISA session"=w733:refnum<visa-resource-name>, "error out"=w732:errorcluster)  [unwired: 15 in]
          }
          frame #3 {
            n118 = local read "Input Mode"() -> (w752:i32)
            n119 = call "SR51XX Configure Sensitivity"("VISA session (for class)"=w756, "Input Mode"=w752, "Range"="Range", "error in (no error)"=w754, "Auto Sensitivity"="Auto Sensitivity", "Auto Measure"="Auto Measure", "Update"=w751) -> ("Range Annotations Out[]"=w745:string[], "VISA session"=w755:refnum<visa-resource-name>, "Auto Sensitivity out"=w748:bool, "Auto Measure out"=w747:bool, "Range Out"=w746:u8, "error out"=w753:errorcluster)  [unwired: 7 in]
            n120 = property on="Range" class="Ring (strict)"("Strings []"=w745) -> ()  [unwired: 2 in, 2 out]
            n121 = local write "Auto Sensitivity"(w748) -> ()
            n122 = local write "Auto Measure"(w747) -> ()
            n123 = local write "Range"(w746) -> ()
          }
          frame #4 {
            n124 = property on="prev_range" class="DigNum (strict)"() -> ("Value"=w760:i32)  [unwired: 2 in, 2 out]
            n125 = property on="Range" class="Ring (strict)"() -> ("Value"=w759:u8)  [unwired: 2 in, 2 out]
            n126 = Equal?(x=w759, y=w760) -> (x = y?=w761:bool)
            n127 = case shown="False" w761 {
              tunnel: w758 -> [w767 _]
              frame False {
                n128 = flat-sequence {
                  tunnel: w767 -> [w769]
                  frame #0 {
                    n129 = property on="Range" class="Ring (strict)"() -> ("Value"=w768:u8)  [unwired: 2 in, 2 out]
                    n130 = property on="prev_range" class="DigNum (strict)"("Value"=w768) -> ()  [unwired: 2 in, 2 out]
                  }
                  frame #1 {
                    n131 = call "read_sense.vi"("VISA session (for class)"=w769) -> ("sense"=w771:string)
                    n132 = Concatenate Strings("Sensitivity: " ("string"), w771) -> (w770:string)
                    n133 = local read "FILE"() -> (w774:refnum<file>)
                    n134 = Format Into String(format string="# %-s\\n", initial string=w774, w770) -> ()  [unwired: 1 in, 2 out]
                  }
                }
              }
              frame True {
              }
            }
          }
          frame #5 {
            n135 = Or(x=w788, y=w787) -> (x .or. y?=w786:bool)
            n136 = call "SR51XX Configure Output Channels - Slope, TC and Dyn Reserve"("VISA session (for class)"=w785, "Time Constant"="Time Constant", "Slope"="Slope", "Check TC"=w786, "Dynamic Reserve"="Dynamic Reserve", "error in (no error)"=w783, "Range"=w778, "Update"=w789) -> ("VISA session"=w784:refnum<visa-resource-name>, "Slope Out"=w779:u8, "Time Constant Out"=w780:u16, "error out"=w782:errorcluster)  [unwired: 8 in]
            n137 = local write "Slope"(w779) -> ()
            n138 = local write "Time Constant"(w780) -> ()
          }
          frame #6 {
            n139 = property on="prev_time_const" class="DigNum (strict)"() -> ("Value"=w792:i32)  [unwired: 2 in, 2 out]
            n140 = property on="Time Constant" class="Ring (strict)"() -> ("Value"=w791:u16)  [unwired: 2 in, 2 out]
            n141 = Equal?(x=w791, y=w792) -> (x = y?=w794:bool)
            n142 = case shown="False" w794 {
              tunnel: w793 -> [w802 _]
              frame False {
                n143 = flat-sequence {
                  tunnel: w802 -> [w804]
                  frame #0 {
                    n144 = property on="Time Constant" class="Ring (strict)"() -> ("Value"=w803:u16)  [unwired: 2 in, 2 out]
                    n145 = property on="prev_time_const" class="DigNum (strict)"("Value"=w803) -> ()  [unwired: 2 in, 2 out]
                  }
                  frame #1 {
                    n146 = call "read_time_const.vi"("VISA session (for class)"=w804) -> ("time_const"=w805:string)
                    n147 = Concatenate Strings("Time Constant: " ("string"), w805) -> (w806:string)
                    n148 = local read "FILE"() -> (w809:refnum<file>)
                    n149 = Format Into String(format string="# %-s\\n", initial string=w809, w806) -> ()  [unwired: 1 in, 2 out]
                  }
                }
              }
              frame True {
              }
            }
          }
          frame #7 {
            n150 = local read "Input Mode"() -> (w823:i32)
            n151 = call "SR5110 Read Output"("VISA session (for class)"=w822, "Input Mode"=w823, "Time Constant"=w819, "Display Type"="Display Type", "Range"=w818, "error in (no error)"=w817, "Slope"=w824) -> ("Units"=→"Units":string, "Display Precision"=w815:i32, "Display"=→"Display":dbl, "VISA session"=w821:refnum<visa-resource-name>, "Available Display Types Out"=w814:string[], "Overload"=→"Overload":bool, "error out"=w816:errorcluster)  [unwired: 4 in, 2 out]
            n152 = property on="Display Type" class="Ring (strict)"("Strings []"=w814) -> ()  [unwired: 2 in, 2 out]
            n153 = property on="Display" class="DigNum (strict)"("Precision"=w815) -> ()  [unwired: 2 in, 2 out]
          }
          frame #8 {
            n154 = local read "Input Mode"() -> (w839:i32)
            n155 = call "SR5110 Read Output"("VISA session (for class)"=w843, "Input Mode"=w839, "Time Constant"=w838, "Display Type"="Display Type 2", "Range"=w836, "error in (no error)"=w842, "Slope"=w835) -> ("Units"=w829:string, "Display Precision"=w833:i32, "Display"=w830:dbl, "VISA session"=w840:refnum<visa-resource-name>, "Available Display Types Out"=w834:string[], "error out"=w841:errorcluster)  [unwired: 4 in, 3 out]
            "Display 2" <- w830
            "Units 2" <- w829
            n156 = call "pref_to_num.vi"("string"=w829) -> ("Numeric"=w832:dbl)
            n157 = property on="Display Type 2" class="Ring (strict)"("Strings []"=w834) -> ()  [unwired: 2 in, 2 out]
            n158 = property on="Display 2" class="DigNum (strict)"("Precision"=w833) -> ()  [unwired: 2 in, 2 out]
            n159 = Multiply(x=w832, y=w830) -> (x*y=w831:dbl)
          }
          frame #9 {
            n160 = local read "Input Mode"() -> (w858:i32)
            n161 = call "SR5110 Read Output"("VISA session (for class)"=w862, "Input Mode"=w858, "Time Constant"=w857, "Display Type"="Display Type 3", "Range"=w855, "error in (no error)"=w860, "Slope"=w854) -> ("Units"=w849:string, "Display Precision"=w853:i32, "Display"=w848:dbl, "VISA session"=w861:refnum<visa-resource-name>, "Available Display Types Out"=w852:string[], "error out"=w859:errorcluster)  [unwired: 4 in, 3 out]
            "Display 3" <- w848
            "Units 3" <- w849
            n162 = property on="Display 3" class="DigNum (strict)"("Precision"=w853) -> ()  [unwired: 2 in, 2 out]
            n163 = call "pref_to_num.vi"("string"=w849) -> ("Numeric"=w851:dbl)
            n164 = property on="Display Type 3" class="Ring (strict)"("Strings []"=w852) -> ()  [unwired: 2 in, 2 out]
            n165 = Multiply(x=w851, y=w848) -> (x*y=w850:dbl)
          }
          frame #10 {
            n166 = local read "Input Mode"() -> (w881:i32)
            n167 = call "SR5110 Read Output"("VISA session (for class)"=w873, "Input Mode"=w881, "Time Constant"=w876, "Display Type"="Display Type copy", "Range"=w875, "error in (no error)"=w874, "Slope"=w877) -> ("Units"=→"Units copy":string, "Display Precision"=w878:i32, "Display"=→"Display copy":dbl, "VISA session"=w868:refnum<visa-resource-name>, "Reference Unlock"=w872:bool, "Available Display Types Out"=w879:string[], "error out"=w869:errorcluster)  [unwired: 4 in, 2 out]
            n168 = property on="Display Type copy" class="Ring (strict)"("Strings []"=w879) -> ()  [unwired: 2 in, 2 out]
            n169 = property on="Display copy" class="DigNum (strict)"("Precision"=w878) -> ()  [unwired: 2 in, 2 out]
            n170 = Bundle By Name(cluster=w867, "5110"=w868, "5110_error_out"=w869) -> (w866:T9)
          }
          frame #11 {
            n171 = local read "Step  (A)"() -> (w891:dbl)
            n172 = local read "Real start cur"() -> (w892:dbl)
            n173 = local read "Real stop cur"() -> (w888:dbl)
            n174 = Multiply(x=w891, y=w890) -> (x*y=w889:dbl)
            n175 = Add(x=w892, y=w889) -> (x+y=w886:dbl)
            n176 = Greater Or Equal?(x=w886, y=w888) -> (x >= y?=w887:bool)
          }
          frame #12 {
            n177 = Unbundle By Name(w896) -> ("6221"=w897:refnum<visa-resource-name>, "6221_error_out"=w898:errorcluster)
            n178 = call <instrlib>:"KE622x -- Set Current Level.vi"("Resource In"=w897, "Current Level (A) In"=w900, "error in (no error)"=w898) -> ("Resource Out (dupl)"=w895:refnum<visa-resource-name>, "error out"=w894:errorcluster)  [unwired: 11 in]
            n179 = Bundle By Name(cluster=w896, "6221"=w895, "6221_error_out"=w894) -> (w893:T9)
            n180 = Wait Until Next ms Multiple(millisecond multiple=u32 50) -> ()  [unwired: 1 out]
          }
          frame #13 {
            n181 = Unbundle By Name(w906) -> ("2000"=w907:refnum<visa-resource-name>, "2000_error_out"=w908:errorcluster, "DAQ_clust.Actual Number of Channels"=w910:u32, "DAQ_clust.Task out"=w909:i32, "DAQ_clust.error out"=w911:errorcluster)
            n182 = call <instrlib>:"Data Read Single.vi"("VISA resource name"=w907, "error in (no error)"=w908) -> ("VISA resource name out"=w903:refnum<visa-resource-name>, "Measurement"=w933:dbl, "error out"=w902:errorcluster)  [unwired: 13 in, 2 out]
            n183 = call-poly <userlib>:"DtOLRead.vi"("Number Chan to Read"=w910, "error in (no error)"=w911, "Task in"=w909) -> ("error out"=w904:errorcluster, "2D Data out"=w927:dbl[][], "Task out"=w905:i32)  [unwired: 4 in, 2 out]
            n184 = Index Array(array=w927, index (row) #1=0 ("index (row)"), index (row) #2=1 ("index (row)"), index (row) #3=2 ("index (row)"), index (row) #4=3 ("index (row)"), index (row) #5=4 ("index (row)")) -> (element #1=w926:dbl[], element #2=w920:dbl[], element #3=w919:dbl[], element #4=w918:dbl[], element #5=w917:dbl[])  [unwired: 5 in]
            n185 = Bundle By Name(cluster=w906, "2000"=w903, "2000_error_out"=w902, "DAQ_clust.Task out"=w905, "DAQ_clust.error out"=w904) -> (w901:T9)
            n186 = Index Array(array=w917, index=0) -> (element=w928:dbl)
            n187 = Index Array(array=w926, index=0) -> (element=w931:dbl)
            n188 = Index Array(array=w920, index=0) -> (element=w932:dbl)
            n189 = Index Array(array=w919, index=0) -> (element=w930:dbl)
            n190 = Index Array(array=w918, index=0) -> (element=w929:dbl)
          }
        }
        n191 = local read "T0"() -> (w399:u32)
        n192 = Subtract(x=w388, y=w399) -> (x-y=w204:u32)
        n193 = Bundle(w372, w308, w309) -> (w263:cluster{dbl, dbl, dbl})  [unwired: 1 in]
        n194 = Bundle(w347, w346, w345, w344, w343, "Measurement"=w342) -> (w348:T10)  [unwired: 1 in]
        n195 = Unbundle(w348) -> (w221:dbl, w220:dbl, w219:dbl, w218:dbl, w217:dbl, "Measurement"=w222:dbl)
        n196 = Unbundle(w263) -> (w225:dbl, w224:dbl, w223:dbl)
        n197 = local read "FILE"() -> (w257:refnum<file>)
        n198 = Unbundle(w348) -> (w297:dbl, w291:dbl, w206:dbl, w283:dbl, w278:dbl, "Measurement"=w300:dbl)
        n199 = Format Into String(format string="%08d  %8.2e %12g %14.5e %12.4e %12.4e  %12.4e %12.4e  %12.4e  %12g \\n", initial string=w257, w204, w225, w222, w224, w223, w221, w220, w219, w218, w217) -> ()  [unwired: 1 in, 2 out]
        n200 = Unbundle(w263) -> (w305:dbl, w273:dbl, w268:dbl)
        n201 = Unbundle(w203) -> (w202:dbl[], w201:dbl[], w200:dbl[], w199:dbl[], w198:dbl[], w197:dbl[], w196:dbl[], w195:dbl[], w194:dbl[], w193:dbl[])
        n202 = Multiply(x=w305, y="Current") -> (x*y=w304:dbl)
        n203 = Divide(x=w204, y=u32 1000) -> (x/y=w373:dbl)
        n204 = Multiply(x=w300, y="2000") -> (x*y=w298:dbl)
        n205 = Multiply(x=w297, y="DAQ A0") -> (x*y=w296:dbl)
        n206 = Multiply(x=w291, y="DAQ A1") -> (x*y=w292:dbl)
        n207 = Multiply(x=w206, y="DAQ A2") -> (x*y=w287:dbl)
        n208 = Multiply(x=w283, y="DAQ A3") -> (x*y=w284:dbl)
        n209 = Multiply(x=w278, y="DAQ A4") -> (x*y=w279:dbl)
        n210 = Multiply(x=w273, y="Lock-In, X") -> (x*y=w274:dbl)
        n211 = Multiply(x=w268, y="Lock-In, Y") -> (x*y=w269:dbl)
        n212 = Build Array (concatenate)(w202, w304) -> (w371:dbl[])
        n213 = Build Array (concatenate)(w201, w373) -> (w370:dbl[])
        n214 = Build Array (concatenate)(w200, w298) -> (w369:dbl[])
        n215 = Build Array (concatenate)(w199, w296) -> (w368:dbl[])
        n216 = Build Array (concatenate)(w198, w292) -> (w367:dbl[])
        n217 = Build Array (concatenate)(w197, w287) -> (w366:dbl[])
        n218 = Build Array (concatenate)(w196, w284) -> (w365:dbl[])
        n219 = Build Array (concatenate)(w195, w279) -> (w339:dbl[])
        n220 = Build Array (concatenate)(w194, w274) -> (w341:dbl[])
        n221 = Build Array (concatenate)(w193, w269) -> (w340:dbl[])
        n222 = Bundle(w371, w370, w369, w368, w367, w366, w365, w339, w341, w340) -> (w358:T8)  [unwired: 1 in]
        n223 = Unbundle(w358) -> (w306:dbl[], w266:dbl[], w303:dbl[], w294:dbl[], w289:dbl[], w286:dbl[], w281:dbl[], w275:dbl[], w271:dbl[], w265:dbl[])
        n224 = property on="TIME GRAPH" class="XYGraph (strict)"("XScale.Mapping Mode"="TIME GRAPH X", "YScale.Mapping Mode"="TIME GRAPH Y") -> ()  [unwired: 2 in, 2 out]
        n225 = Bundle(w266, w306) -> (w307:cluster{dbl[], dbl[]})  [unwired: 1 in]
        n226 = Bundle(w266, w303) -> (w302:cluster{dbl[], dbl[]})  [unwired: 1 in]
        n227 = Bundle(w266, w294) -> (w293:cluster{dbl[], dbl[]})  [unwired: 1 in]
        n228 = Bundle(w266, w289) -> (w288:cluster{dbl[], dbl[]})  [unwired: 1 in]
        n229 = Bundle(w266, w286) -> (w285:cluster{dbl[], dbl[]})  [unwired: 1 in]
        n230 = Bundle(w266, w281) -> (w280:cluster{dbl[], dbl[]})  [unwired: 1 in]
        n231 = Bundle(w266, w275) -> (w276:cluster{dbl[], dbl[]})  [unwired: 1 in]
        n232 = Bundle(w266, w271) -> (w270:cluster{dbl[], dbl[]})  [unwired: 1 in]
        n233 = Bundle(w266, w265) -> (w264:cluster{dbl[], dbl[]})  [unwired: 1 in]
        n234 = Build Array(w307, w302, w293, w288, w285, w280, w276, w270, w264) -> (→"TIME GRAPH":cluster{dbl[], dbl[]}[])
        n235 = Unbundle(w358) -> (w357:dbl[], w356:dbl[], w355:dbl[], w354:dbl[], w353:dbl[], w352:dbl[], w351:dbl[], w350:dbl[], w334:dbl[])  [unwired: 1 out]
        n236 = case shown="\"V, Keithley DAQ A3\"" "X-Axis" {
          tunnel: [w419 w461 w496 w524 w566 w601 w636 w661 w696] -> w349
          tunnel: w357 -> [w416 w460 w495 w531 w565 w600 w634 w669 w704]
          tunnel: w356 -> [w433 w451 w494 w530 w564 w599 w633 w668 w703]
          tunnel: w355 -> [w432 w459 w486 w529 w563 w598 w632 w667 w702]
          tunnel: w354 -> [w431 w458 w493 w521 w562 w597 w631 w666 w701]
          tunnel: w353 -> [w430 w457 w492 w528 w556 w596 w630 w665 w700]
          tunnel: w352 -> [w429 w456 w491 w527 w561 w591 w629 w664 w699]
          tunnel: w351 -> [w428 w455 w490 w526 w560 w595 w635 w663 w698]
          tunnel: w350 -> [w427 w454 w489 w525 w559 w594 w628 w670 w697]
          tunnel: w334 -> [w417 w452 w487 w522 w557 w592 w627 w662 w705]
          frame "I, Keithley 6221", Default {
            n237 = Bundle(w416, w433) -> (w426:cluster{dbl[], dbl[]})  [unwired: 1 in]
            n238 = Bundle(w416, w432) -> (w425:cluster{dbl[], dbl[]})  [unwired: 1 in]
            n239 = Bundle(w416, w431) -> (w424:cluster{dbl[], dbl[]})  [unwired: 1 in]
            n240 = Bundle(w416, w430) -> (w423:cluster{dbl[], dbl[]})  [unwired: 1 in]
            n241 = Bundle(w416, w429) -> (w422:cluster{dbl[], dbl[]})  [unwired: 1 in]
            n242 = Bundle(w416, w428) -> (w421:cluster{dbl[], dbl[]})  [unwired: 1 in]
            n243 = Bundle(w416, w427) -> (w420:cluster{dbl[], dbl[]})  [unwired: 1 in]
            n244 = Bundle(w416, w417) -> (w418:cluster{dbl[], dbl[]})  [unwired: 1 in]
            n245 = Build Array(w426, w425, w424, w423, w422, w421, w420, w418) -> (w419:cluster{dbl[], dbl[]}[])
            n246 = property on="MULTIPLE GRAPHS" class="XYGraph (strict)"("XScale.NameLbl.Text"="Keithley 6221, mA" ("X Scale.Name Label.Text")) -> ()  [unwired: 2 in, 2 out]
            n247 = property on="MULTIPLE GRAPHS" class="XYGraph (strict)"("Active Plot"=u32 0, "Plot.Plot Name"="Mult, 2000 V", "Active Plot"=u32 1, "Plot.Plot Name"="DAQ A0", "Active Plot"=u32 2, "Plot.Plot Name"="DAQ A1", "Active Plot"=u32 3, "Plot.Plot Name"="DAQ A2", "Active Plot"=u32 4, "Plot.Plot Name"="DAQ A3", "Active Plot"=u32 5, "Plot.Plot Name"="DAQ A4", "Active Plot"=u32 6, "Plot.Plot Name"="Lock-In, X", "Active Plot"=u32 7, "Plot.Plot Name"="Lock-In, Y") -> ()  [unwired: 2 in, 2 out]
          }
          frame "V, Keithley 2000" {
            n248 = property on="MULTIPLE GRAPHS" class="XYGraph (strict)"("XScale.NameLbl.Text"="Keithley 2000, V" ("X Scale.Name Label.Text")) -> ()  [unwired: 2 in, 2 out]
            n249 = Bundle(w451, w460) -> (w468:cluster{dbl[], dbl[]})  [unwired: 1 in]
            n250 = Bundle(w451, w459) -> (w467:cluster{dbl[], dbl[]})  [unwired: 1 in]
            n251 = Bundle(w451, w458) -> (w466:cluster{dbl[], dbl[]})  [unwired: 1 in]
            n252 = Bundle(w451, w457) -> (w465:cluster{dbl[], dbl[]})  [unwired: 1 in]
            n253 = Bundle(w451, w456) -> (w464:cluster{dbl[], dbl[]})  [unwired: 1 in]
            n254 = Bundle(w451, w455) -> (w463:cluster{dbl[], dbl[]})  [unwired: 1 in]
            n255 = Bundle(w451, w454) -> (w462:cluster{dbl[], dbl[]})  [unwired: 1 in]
            n256 = Bundle(w451, w452) -> (w453:cluster{dbl[], dbl[]})  [unwired: 1 in]
            n257 = Build Array(w468, w467, w466, w465, w464, w463, w462, w453) -> (w461:cluster{dbl[], dbl[]}[])
            n258 = property on="MULTIPLE GRAPHS" class="XYGraph (strict)"("Active Plot"=u32 0, "Plot.Plot Name"="I, 6221 mA", "Active Plot"=u32 1, "Plot.Plot Name"="DAQ A0", "Active Plot"=u32 2, "Plot.Plot Name"="DAQ A1", "Active Plot"=u32 3, "Plot.Plot Name"="DAQ A2", "Active Plot"=u32 4, "Plot.Plot Name"="DAQ A3", "Active Plot"=u32 5, "Plot.Plot Name"="DAQ A4", "Active Plot"=u32 6, "Plot.Plot Name"="Lock-In, X", "Active Plot"=u32 7, "Plot.Plot Name"="Lock-In, Y") -> ()  [unwired: 2 in, 2 out]
          }
          frame "V, Keithley DAQ A0" {
            n259 = property on="MULTIPLE GRAPHS" class="XYGraph (strict)"("XScale.NameLbl.Text"="Keithley DAQ A0, V" ("X Scale.Name Label.Text")) -> ()  [unwired: 2 in, 2 out]
            n260 = Bundle(w486, w487) -> (w488:cluster{dbl[], dbl[]})  [unwired: 1 in]
            n261 = Bundle(w486, w495) -> (w503:cluster{dbl[], dbl[]})  [unwired: 1 in]
            n262 = Bundle(w486, w494) -> (w502:cluster{dbl[], dbl[]})  [unwired: 1 in]
            n263 = Bundle(w486, w493) -> (w501:cluster{dbl[], dbl[]})  [unwired: 1 in]
            n264 = Bundle(w486, w492) -> (w500:cluster{dbl[], dbl[]})  [unwired: 1 in]
            n265 = Bundle(w486, w491) -> (w499:cluster{dbl[], dbl[]})  [unwired: 1 in]
            n266 = Bundle(w486, w490) -> (w498:cluster{dbl[], dbl[]})  [unwired: 1 in]
            n267 = Bundle(w486, w489) -> (w497:cluster{dbl[], dbl[]})  [unwired: 1 in]
            n268 = Build Array(w503, w502, w501, w500, w499, w498, w497, w488) -> (w496:cluster{dbl[], dbl[]}[])
            n269 = property on="MULTIPLE GRAPHS" class="XYGraph (strict)"("Active Plot"=u32 0, "Plot.Plot Name"="I, 6221 mA", "Active Plot"=u32 1, "Plot.Plot Name"="Mult, 2000 V", "Active Plot"=u32 2, "Plot.Plot Name"="DAQ A1", "Active Plot"=u32 3, "Plot.Plot Name"="DAQ A2", "Active Plot"=u32 4, "Plot.Plot Name"="DAQ A3", "Active Plot"=u32 5, "Plot.Plot Name"="DAQ A4", "Active Plot"=u32 6, "Plot.Plot Name"="Lock-In, X", "Active Plot"=u32 7, "Plot.Plot Name"="Lock-In, Y") -> ()  [unwired: 2 in, 2 out]
          }
          frame "V, Keithley DAQ A1" {
            n270 = property on="MULTIPLE GRAPHS" class="XYGraph (strict)"("XScale.NameLbl.Text"="Keithley DAQ A1, V" ("X Scale.Name Label.Text")) -> ()  [unwired: 2 in, 2 out]
            n271 = Bundle(w521, w531) -> (w533:cluster{dbl[], dbl[]})  [unwired: 1 in]
            n272 = Bundle(w521, w530) -> (w534:cluster{dbl[], dbl[]})  [unwired: 1 in]
            n273 = Bundle(w521, w529) -> (w535:cluster{dbl[], dbl[]})  [unwired: 1 in]
            n274 = Bundle(w521, w528) -> (w536:cluster{dbl[], dbl[]})  [unwired: 1 in]
            n275 = Bundle(w521, w527) -> (w537:cluster{dbl[], dbl[]})  [unwired: 1 in]
            n276 = Bundle(w521, w526) -> (w538:cluster{dbl[], dbl[]})  [unwired: 1 in]
            n277 = Bundle(w521, w525) -> (w539:cluster{dbl[], dbl[]})  [unwired: 1 in]
            n278 = Bundle(w521, w522) -> (w523:cluster{dbl[], dbl[]})  [unwired: 1 in]
            n279 = Build Array(w533, w534, w535, w536, w537, w538, w539, w523) -> (w524:cluster{dbl[], dbl[]}[])
            n280 = property on="MULTIPLE GRAPHS" class="XYGraph (strict)"("Active Plot"=u32 0, "Plot.Plot Name"="I, 6221 mA", "Active Plot"=u32 1, "Plot.Plot Name"="Mult, 2000 V", "Active Plot"=u32 2, "Plot.Plot Name"="DAQ A0", "Active Plot"=u32 3, "Plot.Plot Name"="DAQ A2", "Active Plot"=u32 4, "Plot.Plot Name"="DAQ A3", "Active Plot"=u32 5, "Plot.Plot Name"="DAQ A4", "Active Plot"=u32 6, "Plot.Plot Name"="Lock-In, X", "Active Plot"=u32 7, "Plot.Plot Name"="Lock-In, Y") -> ()  [unwired: 2 in, 2 out]
          }
          frame "V, Keithley DAQ A2" {
            n281 = property on="MULTIPLE GRAPHS" class="XYGraph (strict)"("XScale.NameLbl.Text"="Keithley DAQ A2, V" ("X Scale.Name Label.Text")) -> ()  [unwired: 2 in, 2 out]
            n282 = Bundle(w556, w565) -> (w567:cluster{dbl[], dbl[]})  [unwired: 1 in]
            n283 = Bundle(w556, w564) -> (w568:cluster{dbl[], dbl[]})  [unwired: 1 in]
            n284 = Bundle(w556, w563) -> (w569:cluster{dbl[], dbl[]})  [unwired: 1 in]
            n285 = Bundle(w556, w562) -> (w570:cluster{dbl[], dbl[]})  [unwired: 1 in]
            n286 = Bundle(w556, w561) -> (w571:cluster{dbl[], dbl[]})  [unwired: 1 in]
            n287 = Bundle(w556, w560) -> (w572:cluster{dbl[], dbl[]})  [unwired: 1 in]
            n288 = Bundle(w556, w559) -> (w573:cluster{dbl[], dbl[]})  [unwired: 1 in]
            n289 = Bundle(w556, w557) -> (w558:cluster{dbl[], dbl[]})  [unwired: 1 in]
            n290 = Build Array(w567, w568, w569, w570, w571, w572, w573, w558) -> (w566:cluster{dbl[], dbl[]}[])
            n291 = property on="MULTIPLE GRAPHS" class="XYGraph (strict)"("Active Plot"=u32 0, "Plot.Plot Name"="I, 6221 mA", "Active Plot"=u32 1, "Plot.Plot Name"="Mult, 2000 V", "Active Plot"=u32 2, "Plot.Plot Name"="DAQ A0", "Active Plot"=u32 3, "Plot.Plot Name"="DAQ A1", "Active Plot"=u32 4, "Plot.Plot Name"="DAQ A3", "Active Plot"=u32 5, "Plot.Plot Name"="DAQ A4", "Active Plot"=u32 6, "Plot.Plot Name"="Lock-In, X", "Active Plot"=u32 7, "Plot.Plot Name"="Lock-In, Y") -> ()  [unwired: 2 in, 2 out]
          }
          frame "V, Keithley DAQ A3" {
            n292 = property on="MULTIPLE GRAPHS" class="XYGraph (strict)"("XScale.NameLbl.Text"="Keithley DAQ A3, V" ("X Scale.Name Label.Text")) -> ()  [unwired: 2 in, 2 out]
            n293 = Bundle(w591, w600) -> (w602:cluster{dbl[], dbl[]})  [unwired: 1 in]
            n294 = Bundle(w591, w599) -> (w603:cluster{dbl[], dbl[]})  [unwired: 1 in]
            n295 = Bundle(w591, w598) -> (w604:cluster{dbl[], dbl[]})  [unwired: 1 in]
            n296 = Bundle(w591, w597) -> (w605:cluster{dbl[], dbl[]})  [unwired: 1 in]
            n297 = Bundle(w591, w596) -> (w606:cluster{dbl[], dbl[]})  [unwired: 1 in]
            n298 = Bundle(w591, w595) -> (w607:cluster{dbl[], dbl[]})  [unwired: 1 in]
            n299 = Bundle(w591, w594) -> (w608:cluster{dbl[], dbl[]})  [unwired: 1 in]
            n300 = Bundle(w591, w592) -> (w593:cluster{dbl[], dbl[]})  [unwired: 1 in]
            n301 = Build Array(w602, w603, w604, w605, w606, w607, w608, w593) -> (w601:cluster{dbl[], dbl[]}[])
            n302 = property on="MULTIPLE GRAPHS" class="XYGraph (strict)"("Active Plot"=u32 0, "Plot.Plot Name"="I, 6221 mA", "Active Plot"=u32 1, "Plot.Plot Name"="Mult, 2000 V", "Active Plot"=u32 2, "Plot.Plot Name"="DAQ A0", "Active Plot"=u32 3, "Plot.Plot Name"="DAQ A1", "Active Plot"=u32 4, "Plot.Plot Name"="DAQ A2", "Active Plot"=u32 5, "Plot.Plot Name"="DAQ A4", "Active Plot"=u32 6, "Plot.Plot Name"="Lock-In, X", "Active Plot"=u32 7, "Plot.Plot Name"="Lock-In,Y") -> ()  [unwired: 2 in, 2 out]
          }
          frame "V, Keithley DAQ A4" {
            n303 = property on="MULTIPLE GRAPHS" class="XYGraph (strict)"("XScale.NameLbl.Text"="Keithley DAQ A4, V" ("X Scale.Name Label.Text")) -> ()  [unwired: 2 in, 2 out]
            n304 = Bundle(w635, w634) -> (w638:cluster{dbl[], dbl[]})  [unwired: 1 in]
            n305 = Bundle(w635, w633) -> (w639:cluster{dbl[], dbl[]})  [unwired: 1 in]
            n306 = Bundle(w635, w632) -> (w640:cluster{dbl[], dbl[]})  [unwired: 1 in]
            n307 = Bundle(w635, w631) -> (w641:cluster{dbl[], dbl[]})  [unwired: 1 in]
            n308 = Bundle(w635, w630) -> (w642:cluster{dbl[], dbl[]})  [unwired: 1 in]
            n309 = Bundle(w635, w629) -> (w643:cluster{dbl[], dbl[]})  [unwired: 1 in]
            n310 = Bundle(w635, w628) -> (w644:cluster{dbl[], dbl[]})  [unwired: 1 in]
            n311 = Bundle(w635, w627) -> (w637:cluster{dbl[], dbl[]})  [unwired: 1 in]
            n312 = Build Array(w638, w639, w640, w641, w642, w643, w644, w637) -> (w636:cluster{dbl[], dbl[]}[])
            n313 = property on="MULTIPLE GRAPHS" class="XYGraph (strict)"("Active Plot"=u32 0, "Plot.Plot Name"="I, 6221 mA", "Active Plot"=u32 1, "Plot.Plot Name"="Mult, 2000 V", "Active Plot"=u32 2, "Plot.Plot Name"="DAQ A0", "Active Plot"=u32 3, "Plot.Plot Name"="DAQ A1", "Active Plot"=u32 4, "Plot.Plot Name"="DAQ A2", "Active Plot"=u32 5, "Plot.Plot Name"="DAQ A3", "Active Plot"=u32 6, "Plot.Plot Name"="Lock-In, X", "Active Plot"=u32 7, "Plot.Plot Name"="Lock-In, Y") -> ()  [unwired: 2 in, 2 out]
          }
          frame "V, Lock-In X" {
            n314 = property on="MULTIPLE GRAPHS" class="XYGraph (strict)"("XScale.NameLbl.Text"="Lock-In X, V" ("X Scale.Name Label.Text")) -> ()  [unwired: 2 in, 2 out]
            n315 = Bundle(w670, w669) -> (w672:cluster{dbl[], dbl[]})  [unwired: 1 in]
            n316 = Bundle(w670, w668) -> (w673:cluster{dbl[], dbl[]})  [unwired: 1 in]
            n317 = Bundle(w670, w667) -> (w674:cluster{dbl[], dbl[]})  [unwired: 1 in]
            n318 = Bundle(w670, w666) -> (w675:cluster{dbl[], dbl[]})  [unwired: 1 in]
            n319 = Bundle(w670, w665) -> (w676:cluster{dbl[], dbl[]})  [unwired: 1 in]
            n320 = Bundle(w670, w664) -> (w677:cluster{dbl[], dbl[]})  [unwired: 1 in]
            n321 = Bundle(w670, w663) -> (w678:cluster{dbl[], dbl[]})  [unwired: 1 in]
            n322 = Bundle(w670, w662) -> (w671:cluster{dbl[], dbl[]})  [unwired: 1 in]
            n323 = Build Array(w672, w673, w674, w675, w676, w677, w678, w671) -> (w661:cluster{dbl[], dbl[]}[])
            n324 = property on="MULTIPLE GRAPHS" class="XYGraph (strict)"("Active Plot"=u32 0, "Plot.Plot Name"="I, 6221 mA", "Active Plot"=u32 1, "Plot.Plot Name"="Mult, 2000 V", "Active Plot"=u32 2, "Plot.Plot Name"="DAQ A0", "Active Plot"=u32 3, "Plot.Plot Name"="DAQ A1", "Active Plot"=u32 4, "Plot.Plot Name"="DAQ A2", "Active Plot"=u32 5, "Plot.Plot Name"="DAQ A3", "Active Plot"=u32 6, "Plot.Plot Name"="DAQ A4", "Active Plot"=u32 7, "Plot.Plot Name"="Lock-In, Y") -> ()  [unwired: 2 in, 2 out]
          }
          frame "V, Lock-In Y" {
            n325 = property on="MULTIPLE GRAPHS" class="XYGraph (strict)"("XScale.NameLbl.Text"="Lock-In Y, V" ("X Scale.Name Label.Text")) -> ()  [unwired: 2 in, 2 out]
            n326 = Bundle(w705, w704) -> (w713:cluster{dbl[], dbl[]})  [unwired: 1 in]
            n327 = Bundle(w705, w703) -> (w712:cluster{dbl[], dbl[]})  [unwired: 1 in]
            n328 = Bundle(w705, w702) -> (w711:cluster{dbl[], dbl[]})  [unwired: 1 in]
            n329 = Bundle(w705, w701) -> (w710:cluster{dbl[], dbl[]})  [unwired: 1 in]
            n330 = Bundle(w705, w700) -> (w709:cluster{dbl[], dbl[]})  [unwired: 1 in]
            n331 = Bundle(w705, w699) -> (w708:cluster{dbl[], dbl[]})  [unwired: 1 in]
            n332 = Bundle(w705, w698) -> (w707:cluster{dbl[], dbl[]})  [unwired: 1 in]
            n333 = Bundle(w705, w697) -> (w706:cluster{dbl[], dbl[]})  [unwired: 1 in]
            n334 = Build Array(w713, w712, w711, w710, w709, w708, w707, w706) -> (w696:cluster{dbl[], dbl[]}[])
            n335 = property on="MULTIPLE GRAPHS" class="XYGraph (strict)"("Active Plot"=u32 0, "Plot.Plot Name"="I, 6221 mA", "Active Plot"=u32 1, "Plot.Plot Name"="Mult, 2000 V", "Active Plot"=u32 2, "Plot.Plot Name"="DAQ A0", "Active Plot"=u32 3, "Plot.Plot Name"="DAQ A1", "Active Plot"=u32 4, "Plot.Plot Name"="DAQ A2", "Active Plot"=u32 5, "Plot.Plot Name"="DAQ A3", "Active Plot"=u32 6, "Plot.Plot Name"="DAQ A4", "Active Plot"=u32 7, "Plot.Plot Name"="Lock-In, X") -> ()  [unwired: 2 in, 2 out]
          }
        }
        "MULTIPLE GRAPHS" <- w349
        n336 = property on="MULTIPLE GRAPHS" class="XYGraph (strict)"("XScale.Mapping Mode"="MULTIPLE GRAPHS X", "YScale.Mapping Mode"="MULTIPLE GRAPHS Y") -> ()  [unwired: 2 in, 2 out]
        n337 = Unbundle(w358) -> (w364:dbl[], w363:dbl[], w362:dbl[], w361:dbl[], w360:dbl[], w359:dbl[], w335:dbl[], w336:dbl[], w337:dbl[], w338:dbl[])
        n338 = Multiply(x="Time Delay", y=u16 1000) -> (x*y=w256:u16)
        n339 = Wait Until Next ms Multiple(millisecond multiple=w256) -> ()  [unwired: 1 out]
        "2000" <- w396
        "DAQ A0" <- w347
        "DAQ A1" <- w346
        "DAQ A2" <- w345
        "DAQ A3" <- w344
        "DAQ A4" <- w343
      }
    }
    frame #7 {
      n340 = stacked-sequence {
        frame #0 {
          w944 = TRUE ("Visible")
          n341 = property on="Slope" class="Ring (strict)"("Visible"=w944) -> ()  [unwired: 2 in, 2 out]
          n342 = property on="Range" class="Ring (strict)"("Visible"=w944) -> ()  [unwired: 2 in, 2 out]
          n343 = property on="Time Constant" class="Ring (strict)"("Visible"=w944) -> ()  [unwired: 2 in, 2 out]
          n344 = property on="Dynamic Reserve" class="Ring (strict)"("Visible"=w944) -> ()  [unwired: 2 in, 2 out]
          n345 = property on="Auto Sensitivity" class="Bool (strict)"("Visible"=w944) -> ()  [unwired: 2 in, 2 out]
          n346 = property on="Auto Measure" class="Bool (strict)"("Visible"=w944) -> ()  [unwired: 2 in, 2 out]
        }
        frame #1 {
          w945 = TRUE ("Visible")
          n347 = property on="Start \ncurrent (A)" class="DigNum (strict)"("Visible"=w945) -> ()  [unwired: 2 in, 2 out]
          n348 = property on="Stop\ncurrent (A)" class="DigNum (strict)"("Visible"=w945) -> ()  [unwired: 2 in, 2 out]
          n349 = property on="LIMIT" class="Bool (strict)"("Visible"=w945) -> ()  [unwired: 2 in, 2 out]
          n350 = property on="LIMIT" class="Bool (strict)"("Visible"=w945) -> ()  [unwired: 2 in, 2 out]
          n351 = property on="Start cur prefix" class="Ring (strict)"("Visible"=w945) -> ()  [unwired: 2 in, 2 out]
          n352 = property on="Stop cur prefix" class="Ring (strict)"("Visible"=w945) -> ()  [unwired: 2 in, 2 out]
          n353 = property on="Step  (A)" class="DigNum (strict)"("Visible"=w945) -> ()  [unwired: 2 in, 2 out]
          n354 = property on="Number \nof points" class="DigNum (strict)"("Visible"=w945) -> ()  [unwired: 2 in, 2 out]
          n355 = property on="Time Delay" class="Ring (strict)"("Visible"=w945) -> ()  [unwired: 2 in, 2 out]
          n356 = property on="Error Code" class="Str"("Visible"=w945) -> ()  [unwired: 2 in, 2 out]
        }
      }
      n357 = Unbundle By Name(w942) -> ("5110"=w941:refnum<visa-resource-name>, "5110_error_out"=w940:errorcluster, "6221"=w939:refnum<visa-resource-name>, "6221_error_out"=w938:errorcluster, "2000"=w937:refnum<visa-resource-name>, "2000_error_out"=w936:errorcluster, "DAQ_clust.Task out"=w935:i32, "DAQ_clust.error out"=w934:errorcluster)
      n358 = call "SR51XX Close"("error in (no error)"=w940, "VISA session"=w941) -> ()  [unwired: 1 out]
      n359 = call <instrlib>:"Close.vi"("VISA resource name"=w939, "error in (no error)"=w938) -> ()  [unwired: 13 in, 1 out]
      n360 = call <instrlib>:"Close.vi"("VISA resource name"=w937, "error in (no error)"=w936) -> ()  [unwired: 17 in, 1 out]
      n361 = call <userlib>:"DtOLCloseTask.vi"("Error in"=w934, "Task in"=w935) -> ("Error Out"=w943:errorcluster)  [unwired: 9 in]
      n362 = call <vilib>:"Simple Error Handler.vi"("error in (no error)"=w943) -> ()  [unwired: 4 in, 5 out]
    }
  }
